vi "CMN_ToServerLogQ.vi"(4 "error in (no error)":errorcluster, 5 "Mode":enum16{"ALL", "DIFF"}(ring), 7 "Log":bool=TRUE, 8 "file":path, 9 "string":string, 10 "type":u16(ring) items=["command", "imediateReply", "Callback Reply", "Information", "none"]) -> (0 "error out":errorcluster)   [LabVIEW 2016]
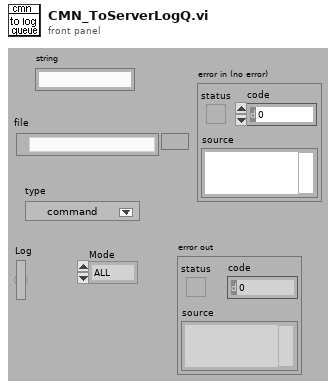
[diagram p1: front panel]
types:
  T1 = cluster{"string":string, "file":path, "type":u16}
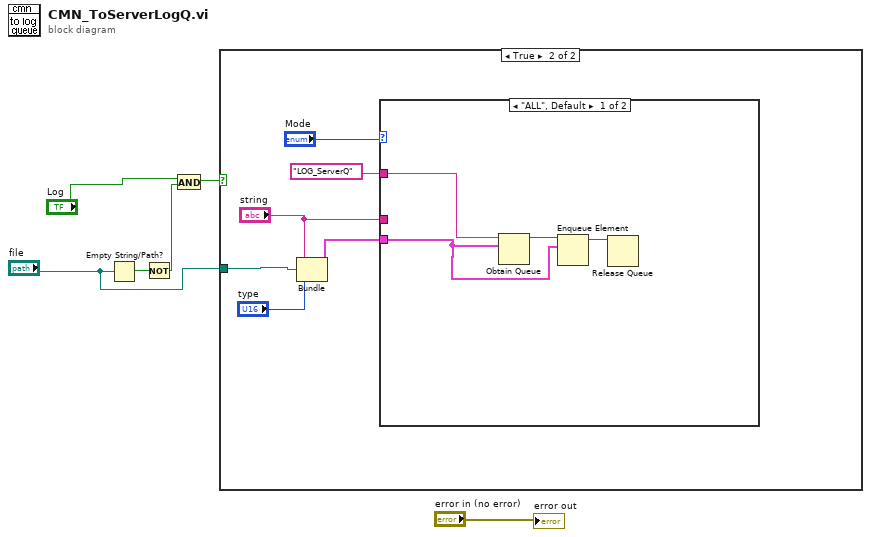
[diagram p0: block diagram]
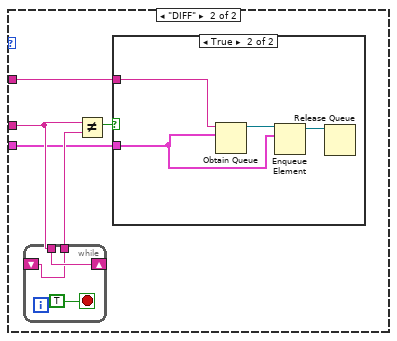
[diagram p3: hidden frame]
diagram:
  n1 = Empty String/Path?(string/path="file") -> (empty?=w5:bool)
  n2 = Not(x=w5) -> (.not. x?=w4:bool)
  n3 = And(x="Log", y=w4) -> (x .and. y?=w3:bool)
  n4 = case shown="True" w3 {
    tunnel: "file" -> [_ w9]
    frame False {
    }
    frame True {
      n5 = Bundle("string"="string", "file"=w9, "type"="type") -> (w8:T1)  [unwired: 1 out]
      n6 = case shown="\"ALL\", Default" "Mode" {
        tunnel: "string" -> [_ w20]
        tunnel: w8 -> [w14 w18]
        tunnel: "LOG_ServerQ" ("name (unnamed)") -> [w13 w17]
        frame "ALL", Default {
          n7 = Obtain Queue(name (unnamed)=w13, element data type=w14) -> (queue out=w16:refnum<queue>)  [unwired: 3 in, 2 out]
          n8 = Enqueue Element(queue=w16, element=w14) -> (queue out=w15:refnum<queue>)  [unwired: 1 in, 3 out]
          n9 = Release Queue(queue=w15) -> ()  [unwired: 1 in, 4 out]
        }
        frame "DIFF" {
          n10 = while {
            tunnel: [w22] -> w19
            tunnel: w20 -> [w23]
            shift-left: _ -> [w22]
            shift-right: [w23] -> _
            stop <- TRUE stop-if-true
          }
          n11 = Not Equal?(x=w20, y=w19) -> (x != y?=w21:bool)
          n12 = case shown="True" w21 {
            tunnel: w18 -> [_ w27]
            tunnel: w17 -> [_ w25]
            frame False {
            }
            frame True {
              n13 = Obtain Queue(name (unnamed)=w25, element data type=w27) -> (queue out=w28:refnum<queue>)  [unwired: 3 in, 2 out]
              n14 = Enqueue Element(queue=w28, element=w27) -> (queue out=w26:refnum<queue>)  [unwired: 1 in, 3 out]
              n15 = Release Queue(queue=w26) -> ()  [unwired: 1 in, 4 out]
            }
          }
        }
      }
    }
  }
  "error out" <- "error in (no error)"
